vi "Update Progress.vi"(8 "error in (no error)":errorcluster, 10 "Glyph":T1, 11 "Message":string) -> (0 "error out":errorcluster)   [LabVIEW 2015, in "Launcher Actor API.lvclass"]
uses:
  Launcher Actor API.lvclass
  Actor/Glyph.ctl
  Actor/Launcher Message.ctl
  Re-use Libraries/Minimal Actor Framework/Messaging/Message/Message.lvclass/Message.ctl
  Globals.vi
  Re-use Libraries/Minimal Actor Framework/Messaging/Message/Message.lvclass
  Re-use Libraries/Minimal Actor Framework/Actors/Base Actor/API/Actor API.lvclass
  Actor/Launcher Actor.lvclass
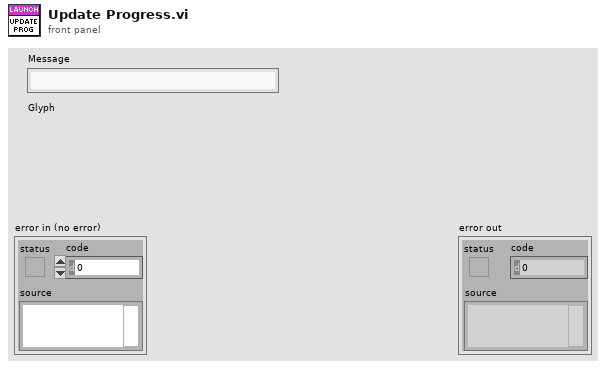
[diagram p1: front panel]
types:
  T1 = typedef "Launcher Actor.lvclass/Glyph.ctl" = u16
  T2 = typedef "Launcher Actor.lvclass/Launcher Message.ctl" = cluster{"Message":string, "Glyph":T1}
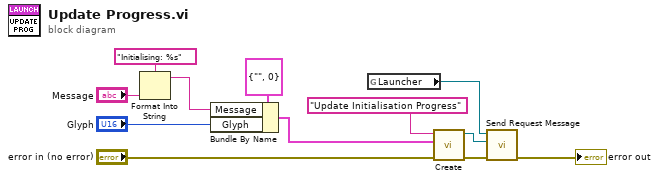
[diagram p0: block diagram]
diagram:
  n1 = Format Into String(format string="Initialising: %s" ("resulting string"), "Message") -> (resulting string=w1:string)  [unwired: 2 in, 1 out]
  n2 = Bundle By Name(cluster=T2 {"Message"="", "Glyph"=0} ("Launcher Message"), "Message"=w1, "Glyph"="Glyph") -> (w2:T2)
  n3 = global read "Globals.vi" "Launcher"() -> (w5:refnum<class "Actor API.lvclass">)
  n4 = call "Create.vi"("error in (no error)"="error in (no error)", "Data"=w2, "Name"="Update Initialisation Progress" ("Parameter")) -> ("error out"=w6:errorcluster, "Message out"=w7:refnum<class "Message.lvclass">)  [unwired: 7 in]
  n5 = call-dynamic "Send Request Message.vi"("error in (no error)"=w6, "Message"=w7, "Actor API in"=w5) -> ("error out"=→"error out":errorcluster)  [unwired: 8 in]
